vi "Unpack.vi"(11 "ClusterMessagePacket":refnum<class "ClusterMessagePacket.lvclass">) -> (3 "Packet":T1)   [LabVIEW 2020, in "Network Messenger.lvlib" / "ClusterMessagePacket.lvclass"]
uses:
  <vilib>/gpm_packages/@cs/Network-interface/Source/Network Messenger/ClusterMessagePacket/ClusterMessagePacket.lvclass
  <vilib>/gpm_packages/@cs/Network-interface/Source/Network Messenger/Types/Message Packet.ctl
  <vilib>/gpm_packages/@cs/Network-interface/Source/Network Messenger/ClusterMessagePacket/ClusterMessagePacket.lvclass/ClusterMessagePacket.ctl
  <vilib>/gpm_packages/@cs/Network-interface/Source/Network Messenger/Network Messenger.lvlib
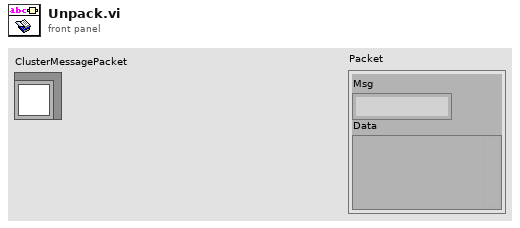
[diagram p1: front panel]
types:
  T1 = typedef "Network Messenger.lvlib/Message Packet.ctl" = cluster{"Msg":string, "Data":variant}
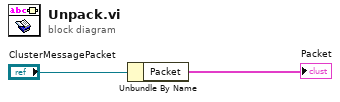
[diagram p0: block diagram]
diagram:
  n1 = Unbundle By Name("ClusterMessagePacket") -> ("Packet"=→"Packet":T1)
